vi "test_output_interpolation.vi"() -> ()   [LabVIEW 2013]
uses:
  <vilib>/rvi/FXPMathLib/FxpConvert/subVIs/nifxpmath_Convert_SimConfig.ctl
  <vilib>/fxp/LVFixedPointQuantizationPolicyTypeDef.ctl
  <vilib>/fxp/LVFixedPointOverflowPolicyTypeDef.ctl
  <vilib>/rvi/FXPMathLib/FxpConvert/simVIs/DllFxpConvertTemp_sub.vi
  <vilib>/rvi/FXPMathLib/FxpInterpret/XNode/nifxpmath_Interpret.xnode
  <vilib>/rvi/FXPMathLib/FxpConvert/XNode/nifxpmath_Convert.xnode
panel:
  out "Waveform Graph 2":i16[](graph)
  out "size(s) 2":i32
  out "size(s)":i32[](array[numeric])
  out "Numeric":i32
  out "Waveform Graph":i16[](graph)
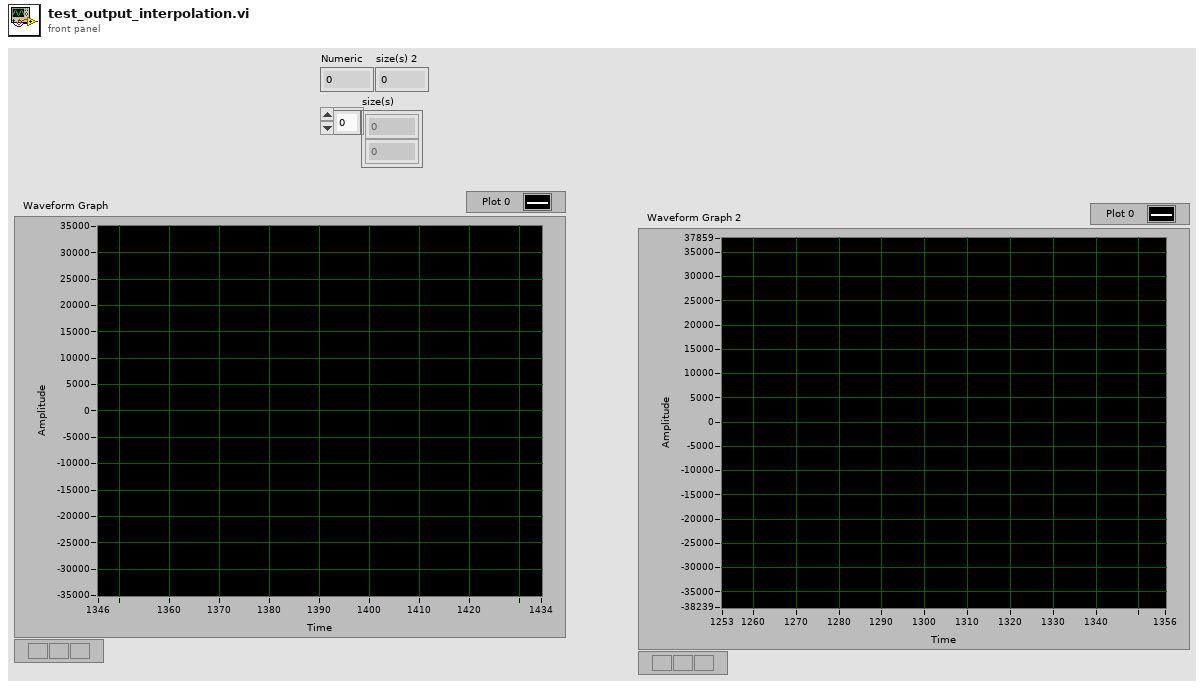
[diagram p1: front panel]
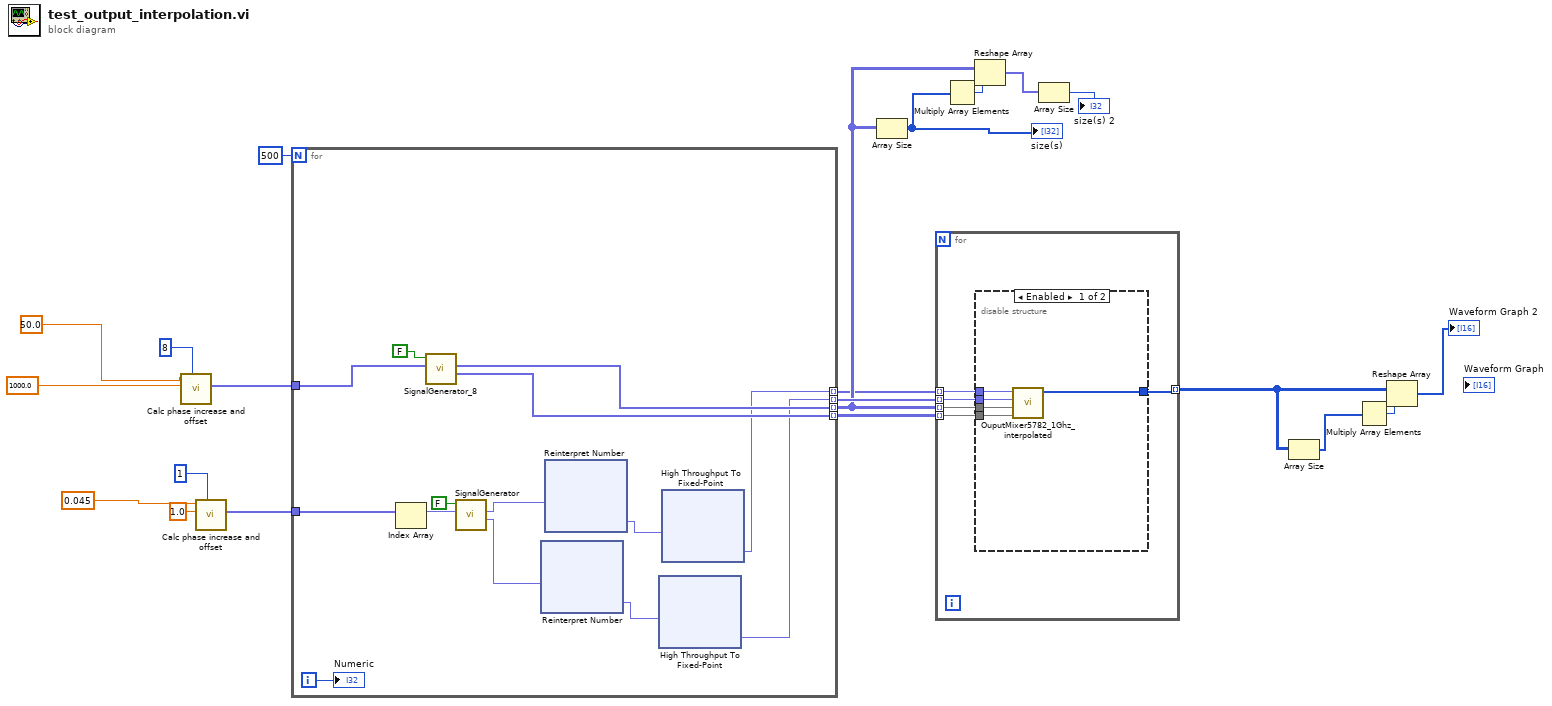
[diagram p0: block diagram]
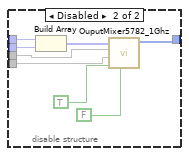
[diagram p2: hidden frame]
diagram:
  n1 = call "Calc phase increase and offset.vi"("# of DDS"=8, "fclk (MHz)"=1000.0 ("fclk (800MHz)"), "f_generated (MHz)"=50.0) -> ("Phase out"=w18:fxp<+,64,64>[])  [unwired: 6 in, 2 out]
  n2 = call "Calc phase increase and offset.vi"("# of DDS"=1, "fclk (MHz)"=1.0, "f_generated (MHz)"=0.045) -> ("Phase out"=w14:fxp<+,64,64>[])  [unwired: 6 in, 2 out]
  n3 = for {
    N: 500 -> [_]
    tunnel: w18 -> [w34]
    tunnel: w14 -> [w33]
    tunnel: [w30] -> w13 mode=indexing
    tunnel: [w27] -> w10 mode=indexing
    tunnel: [w24] -> w2 mode=indexing
    tunnel: [w22] -> w12 mode=indexing
    i -> [w26]
    n4 = Index Array(array=w33) -> (element=w32:fxp<+,64,64>)  [unwired: 1 in]
    n5 = call "SignalGenerator_8.vi"("Phase"=w34, "reset"=FALSE) -> ("Sine out"=w30:fxp<+/-,16,0>[], "Cosine out"=w27:fxp<+/-,16,0>[])  [unwired: 8 in]
    n6 = call "SignalGenerator.vi"("phase"=w32, "Reset"=FALSE) -> ("Cos"=w28:fxp<+/-,16,0>, "Sin"=w29:fxp<+/-,16,0>)  [unwired: 7 in, 1 out]
    n7 = xnode "Reinterpret Number"("x"=w28) -> ("y"=w23:fxp<+/-,16,12>)
    n8 = xnode "Reinterpret Number"("x"=w29) -> ("y"=w25:fxp<+/-,16,12>)
    n9 = xnode "High Throughput To Fixed-Point"("x"=w23) -> ("y"=w22:fxp<+/-,16,14>)
    n10 = xnode "High Throughput To Fixed-Point"("x"=w25) -> ("y"=w24:fxp<+/-,16,14>)
    "Numeric" <- w26
  }
  n11 = Array Size(array=w10) -> (size(s)=w9:i32[])
  "size(s)" <- w9
  n12 = for {
    tunnel: w13 -> [w84] mode=indexing
    tunnel: w10 -> [w83] mode=indexing
    tunnel: w2 -> [w82] mode=indexing
    tunnel: w12 -> [w81] mode=indexing
    tunnel: [w80] -> w3 mode=indexing
    n13 = disable-structure shown="Enabled" {
      disable-tunnel: w84 -> [w89 w92]
      disable-tunnel: w83 -> [w88 w93]
      disable-tunnel: w82 -> [w87 w95]
      disable-tunnel: w81 -> [w86 w96]
      disable-tunnel: [w85 w97] -> w80
      frame Enabled {
        n14 = call "OuputMixer5782_1Ghz_interpolated.vi"("Sine in"=w89, "Cosine in"=w88, "Q"=w86, "I"=w87) -> ("test"=w85:i16[])  [unwired: 7 in]
      }
      frame Disabled {
        n15 = Build Array(w95, w96) -> (w94:fxp<+/-,16,14>[])
        n16 = call "OuputMixer5782_1Ghz.vi"("reset"=FALSE, "valid in"=TRUE, "Sine in"=w92, "Cosine in"=w93, "Data in"=w94) -> ("test"=w97:i16[])  [unwired: 5 in, 1 out]
      }
    }
  }
  n17 = Multiply Array Elements(1:w9) -> (0:w8:i32)
  n18 = Reshape Array(w10, w8) -> (w7:fxp<+/-,16,0>[])
  n19 = Array Size(array=w7) -> (size(s)=→"size(s) 2":i32)
  n20 = Array Size(array=w3) -> (size(s)=w4:i32[])
  n21 = Multiply Array Elements(1:w4) -> (0:w5:i32)
  n22 = Reshape Array(w3, w5) -> (→"Waveform Graph 2":i16[])
